vi "downsample 1D array - U32.vi"(2 "Ave N":dbl, 3 "Array In":i16[](array[numeric])) -> (1 "Array Out":u32[](array[numeric]))   [LabVIEW 2014]
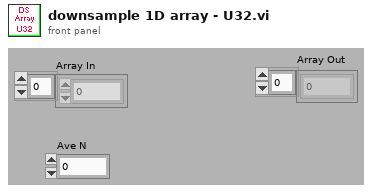
[diagram p1: front panel]
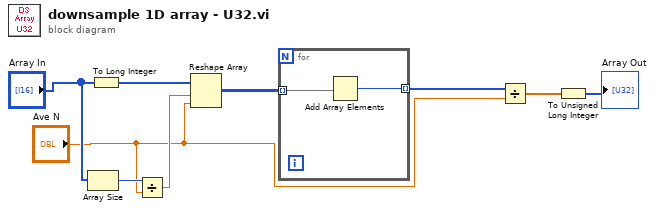
[diagram p0: block diagram]
diagram:
  n1 = Array Size(array="Array In") -> (size(s)=w8:i32)
  n2 = To Long Integer(number="Array In") -> (32bit integer=w4:i32[])
  n3 = Divide(x=w8, y="Ave N") -> (x/y=w6:dbl)
  n4 = Reshape Array(w4, w6, "Ave N") -> (w5:i32[][])
  n5 = for {
    tunnel: w5 -> [w11] mode=indexing
    tunnel: [w10] -> w7 mode=indexing
    n6 = Add Array Elements(numeric array=w11) -> (sum=w10:i32)
  }
  n7 = Divide(x=w7, y="Ave N") -> (x/y=w3:dbl[])
  n8 = To Unsigned Long Integer(number=w3) -> (unsigned 32bit integer=→"Array Out":u32[])
